vi "PPFS_TRAJECTORY_CMD_FIND_FOLLOW_SWERVE.vi"(6 "Pass_Through_Time":dbl=-1.0 format="%33.4f", 8 "Init":bool, 11 "Target Pose M":T1={"TRANSLATION"={"X"=0.0, "Y"=0.0}, "ROTATION"={"VALUE"=0.0, "COS"=1.0, "SIN"=0.0}} {"ROTATION"."SIN" format="%13.4f"; "ROTATION"."COS" format="%13.4f"; "ROTATION"."VALUE" format="%13.4f"; "TRANSLATION"."Y" format="%14.3f"; "TRANSLATION"."X" format="%14.3f"}) -> (0 "AtReference":bool, 1 "Complete":bool, 3 "Chassis Velocity Target SI":T4 {"vOmega" format="%10.3f"; "vY" format="%10.3f"; "vX" format="%10.3f"})   [LabVIEW 2019]
uses:
  <vilib>/Rock Robotics/WPI/ThirdParty/JAS_Junk/TrajLib/Trajectory_Library.lvlib
  PPFS_TRAJECTORY_GLOBALS.vi
  <vilib>/Rock Robotics/WPI/ThirdParty/MJansen/PathPlanner/PathPlanner24.lvlib
  <vilib>/Rock Robotics/WPI/ThirdParty/JAS_Junk/TrajLib/TypeDef/CHASSIS_SPEEDS.ctl
  <vilib>/Rock Robotics/WPI/ThirdParty/JAS_Junk/TrajLib/TypeDef/TRANSLATION2D.ctl
  <vilib>/Rock Robotics/WPI/ThirdParty/JAS_Junk/TrajLib/TypeDef/ROTATION2D.ctl
  <vilib>/Rock Robotics/WPI/ThirdParty/JAS_Junk/TrajLib/TypeDef/POSE2D.ctl
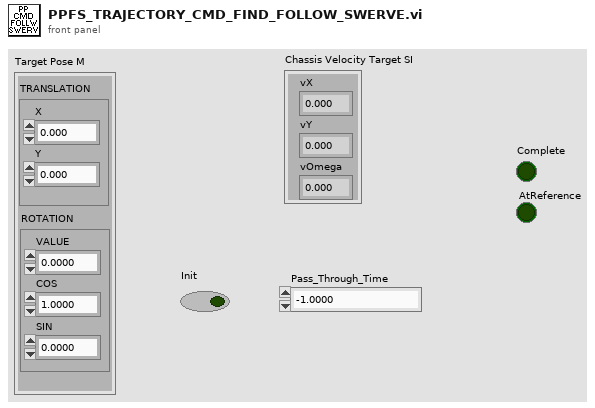
[diagram p1: front panel]
types:
  T1 = typedef "Trajectory_Library.lvlib/POSE2D.ctl" = cluster{"TRANSLATION":T2, "ROTATION":T3}
  T2 = typedef "Trajectory_Library.lvlib/TRANSLATION2D.ctl" = cluster{"X":dbl, "Y":dbl}
  T3 = typedef "Trajectory_Library.lvlib/ROTATION2D.ctl" = cluster{"VALUE":dbl, "COS":dbl, "SIN":dbl}
  T4 = typedef "Trajectory_Library.lvlib/CHASSIS_SPEEDS.ctl" = cluster{"vX":dbl, "vY":dbl, "vOmega":dbl}
  T5 = typedef "PathPlanner24.lvlib/PathPlannerPathConstraints.ctl" = cluster{"MaxVelocityMps;":dbl, "MaxAccelerationMpsSq;":dbl, "MaxAngularVelRadPsEc;":dbl, "MaxAngularAccRadPSecSq":dbl, "Exists":bool}
  T6 = typedef "Trajectory_Library.lvlib/PID_TUNING.ctl" = cluster{"Kp":dbl, "Ki":dbl, "Kd":dbl, "MaximumIntegral":dbl, "MinimumIntegral":dbl}
  T7 = typedef "Trajectory_Library.lvlib/PROFILED_PID_CONTROLLER.ctl" = cluster{"Controller":T8, "Goal":T9, "Setpoint":T9, "Constraint":T10}
  T8 = typedef "Trajectory_Library.lvlib/PID_CONTROLLER.ctl" = cluster{"Kp":dbl, "Ki":dbl, "Kd":dbl, "Period":dbl, "Max_Integral":dbl, "Min_Integral":dbl, "Max_Input":dbl, "Min_Input":dbl, "Continuous":bool, "PositionError":dbl, "VelocityError":dbl, "PrevError":dbl, "TotalError":dbl, "PositionTolerance":dbl, "VelocityTolerance":dbl, "SetPoint":dbl, "Kf":dbl, "Prev_Deriv":dbl, "Prev_Deriv 2":dbl, "DerivativeFilter":bool, "Min_Output":dbl, "Max_Output":dbl, "Prev_F_P":dbl, "Prev_F_P_2":dbl, "AntiWindupActive":bool, "Measurement":dbl}
  T9 = typedef "Trajectory_Library.lvlib/TRAPEZOID_PROFILE_STATE.ctl" = cluster{"Position":dbl, "Velocity":dbl}
  T10 = typedef "Trajectory_Library.lvlib/TRAPEZOID_PROFILE_CONSTRAINT.ctl" = cluster{"MaxVelocity":dbl, "MaxAcceleration":dbl}
  T11 = typedef "PathPlanner24.lvlib/PathPlannerReplanningConfig.ctl" = cluster{"enableInitialReplanning":bool, "enableDynamicReplanning":bool, "dynamicReplanningTotalErrorThreshold":dbl, "dynamicReplanningErrorSpikeThreshold":dbl}
  T12 = typedef "Trajectory_Library.lvlib/HOLONOMIC_PACK_TUNING.ctl" = cluster{"X PID Tuning":T6, "Y PID Tuning":T6, "thetaProfiledPID_CTRL":T7}
  T13 = typedef "PathPlanner24.lvlib/PathPlannerCmdFindConfig.ctl" = cluster{"Goal Position":T2, "GoalEndState":T14, "PathPlannerPathConstraints":T5, "Rotation Delay Distance M":dbl}
  T14 = typedef "PathPlanner24.lvlib/PathPlannerGoalEndState.ctl" = cluster{"Velocity":dbl, "Rotation":T3}
  T15 = typedef "PathPlanner24.lvlib/PathPlannerCmdFollowHolConfig.ctl" = cluster{"HOLONOMIC_CTRL_PACK_TUNING":T12, "Max Wheel Speed M/S":dbl, "Tolerance SI":T1, "Drive Base Radius M":dbl, "ControlPastEnd_Sec":dbl, "ReplanningConfig":T11, "Period_Sec":dbl, "Trigger Events":bool}
  T16 = typedef "Trajectory_Library.lvlib/HOLONOMIC_DRV_CTRL.ctl" = cluster{"poseTolerance":T1, "poseError":T1, "Enabled":bool, "PID_xCtrl":T8, "PID_yCtrl":T8, "PROF_PID_thetaCtrl":T7, "RotationError":T3, "FirstRun":bool}
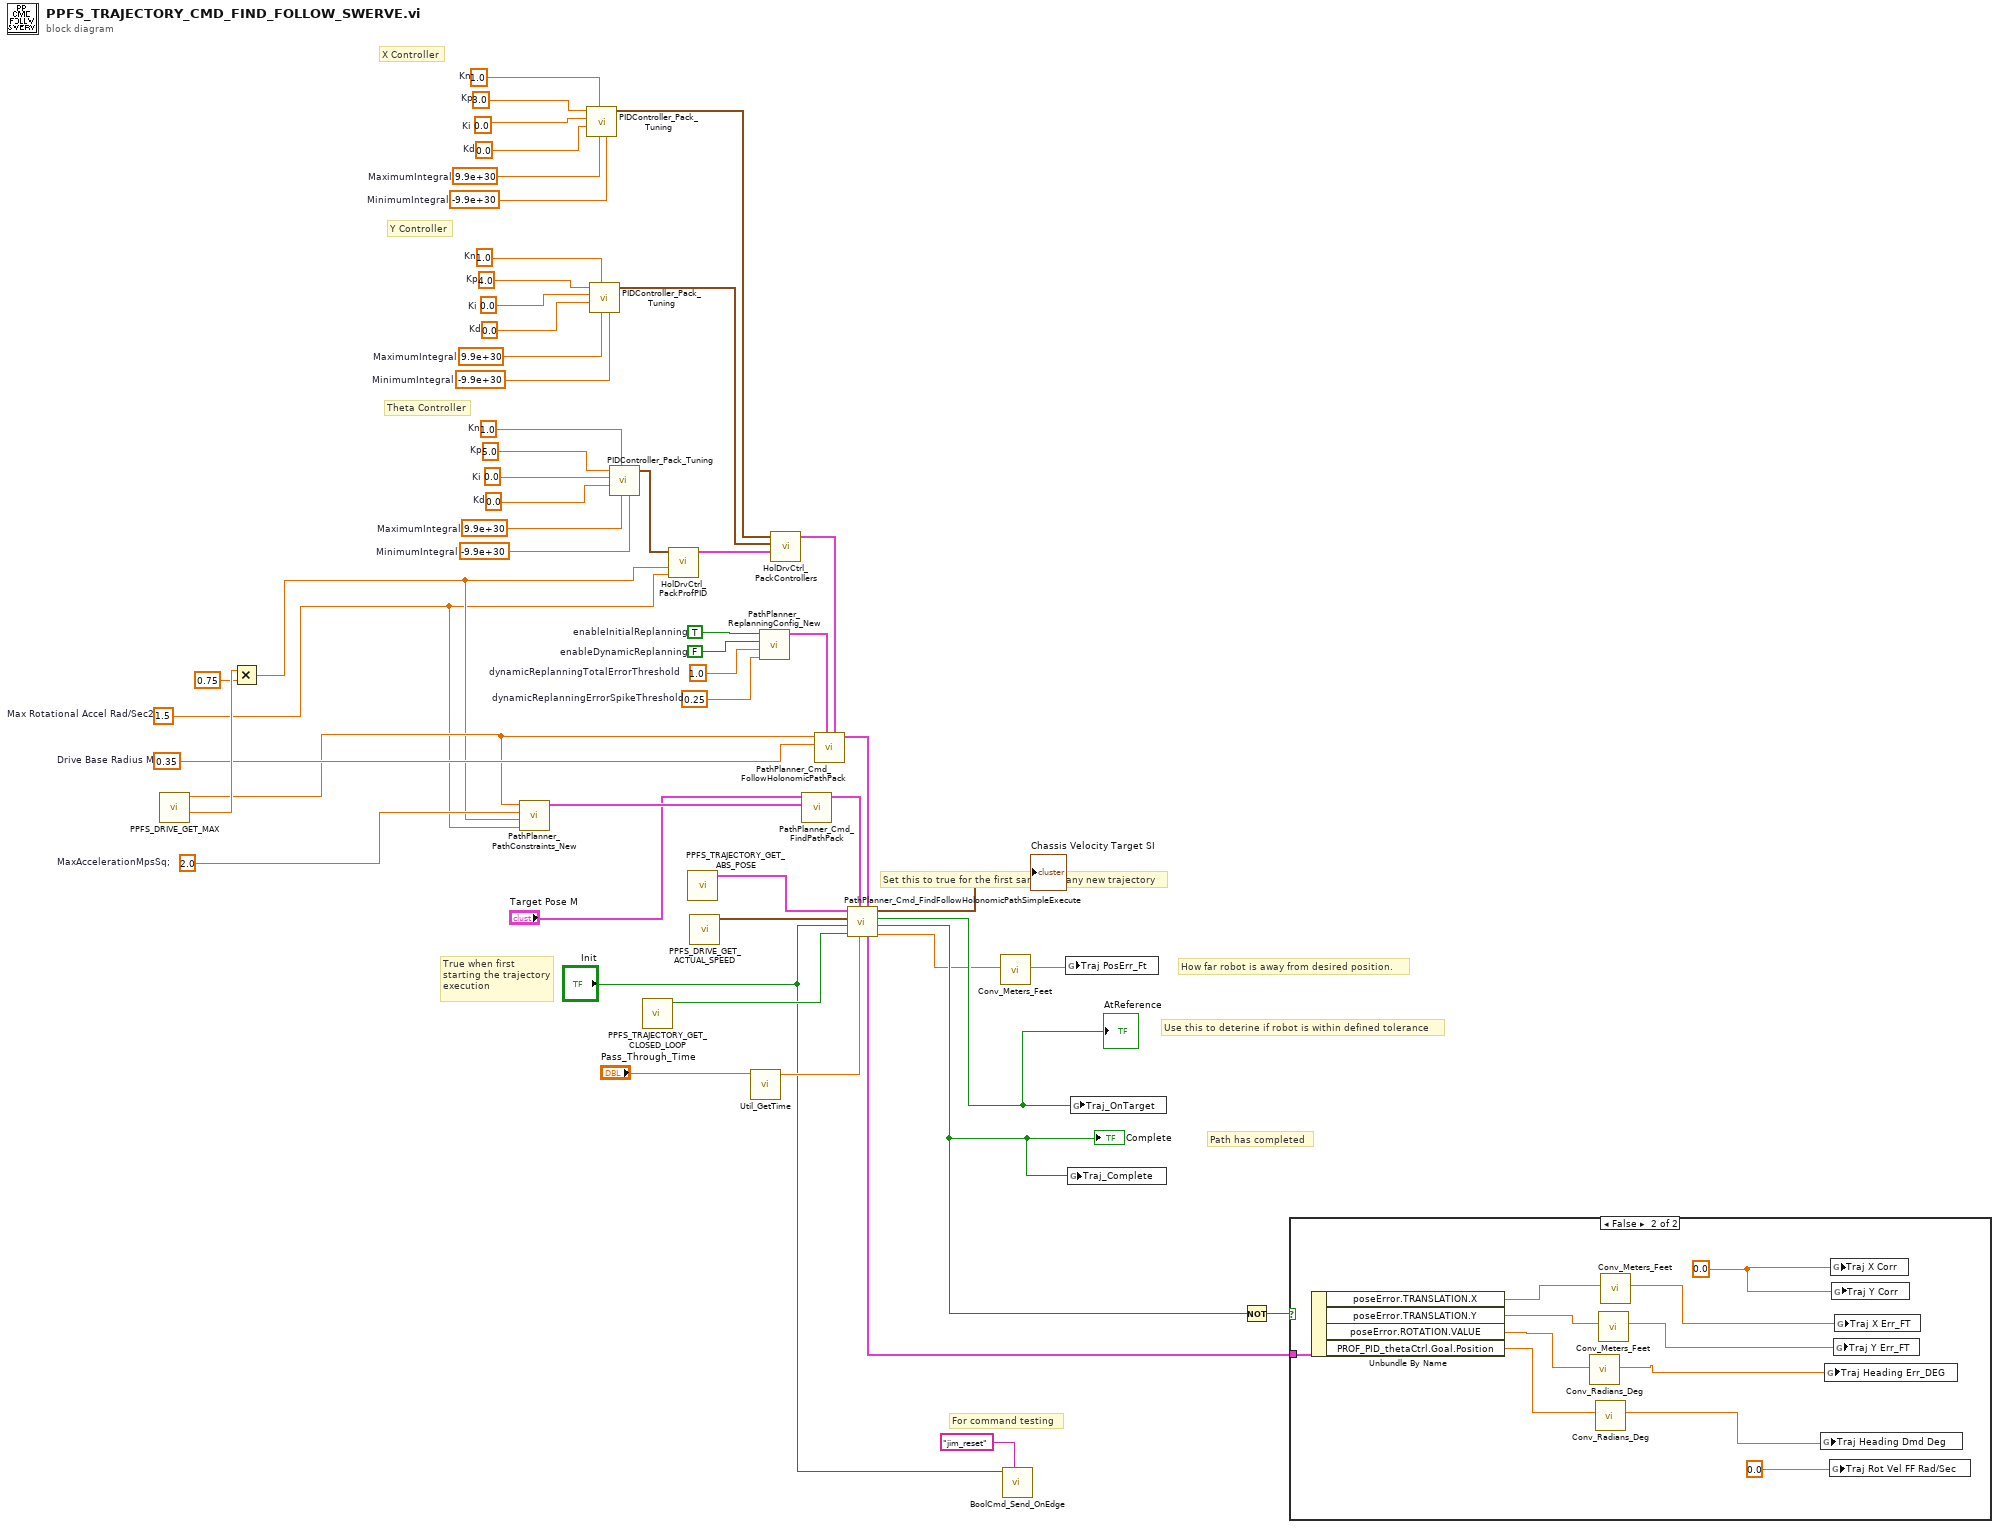
[diagram p0: block diagram]
diagram:
  w6 = 2.0  # MaxAccelerationMpsSq;
  w51 = TRUE  # enableInitialReplanning
  w50 = FALSE  # enableDynamicReplanning
  w49 = 1.0  # dynamicReplanningTotalErrorThreshold
  w48 = 0.25  # dynamicReplanningErrorSpikeThreshold
  w38 = 1.0  # Kn
  w35 = 5.0  # Kp
  w26 = 0.0  # Ki
  w25 = 0.0  # Kd
  w24 = 9.9e+30  # MaximumIntegral
  w23 = -9.9e+30  # MinimumIntegral
  w40 = 1.0  # Kn
  w37 = 3.0  # Kp
  w34 = 0.0  # Ki
  w33 = 0.0  # Kd
  w32 = 9.9e+30  # MaximumIntegral
  w31 = -9.9e+30  # MinimumIntegral
  w39 = 1.0  # Kn
  w36 = 4.0  # Kp
  w30 = 0.0  # Ki
  w29 = 0.0  # Kd
  w28 = 9.9e+30  # MaximumIntegral
  w27 = -9.9e+30  # MinimumIntegral
  w22 = 0.35  # Drive Base Radius M
  w1 = 1.5  # Max Rotational Accel Rad/Sec2
  # "Set this to true for the first sample of any new trajectory"
  # "For command testing"
  # "Path has completed"
  # "How far robot is away from desired position."
  # "Use this to deterine if robot is within defined tolerance"
  # "Theta Controller"
  # "Y Controller"
  # "X Controller"
  # "True when first\nstarting the trajectory\nexecution"
  n1 = call "PPFS_DRIVE_GET_MAX.vi"() -> ("Max Rotational Vel (Rad/Sec)"=w53:dbl, "Max Wheel Vel (Meter/Sec)"=w3:dbl)  [unwired: 10 in]
  n2 = Multiply(x=w53, y=0.75) -> (x*y=w2:dbl)
  n3 = call <vilib>:"PathPlanner_PathConstraints_New.vi"("MaxAngularAccRadPSecSq"=w1, "MaxAngularVelRadPsEc;"=w2, "MaxAccelerationMpsSq;"=w6, "MaxVelocityMps;"=w3) -> ("PathPlannerConstraints"=w7:T5)  [unwired: 7 in]
  n4 = call <vilib>:"PIDController_Pack_Tuning.vi"("MinimumIntegral"=w31, "MaximumIntegral"=w32, "Kn"=w40, "Kd"=w33, "Ki"=w34, "Kp"=w37) -> ("PID Tuning"=w44:T6)  [unwired: 5 in]
  n5 = call <vilib>:"PIDController_Pack_Tuning.vi"("MinimumIntegral"=w27, "MaximumIntegral"=w28, "Kn"=w39, "Kd"=w29, "Ki"=w30, "Kp"=w36) -> ("PID Tuning"=w45:T6)  [unwired: 5 in]
  n6 = call <vilib>:"PIDController_Pack_Tuning.vi"("MinimumIntegral"=w23, "MaximumIntegral"=w24, "Kn"=w38, "Kd"=w25, "Ki"=w26, "Kp"=w35) -> ("PID Tuning"=w41:T6)  [unwired: 5 in]
  n7 = call "PPFS_TRAJECTORY_GET_CLOSED_LOOP.vi"() -> ("AUTO_CLOSED_LOOP"=w19:bool)  [unwired: 11 in]
  n8 = call <vilib>:"HolDrvCtrl_PackProfPID.vi"("Max Accel"=w1, "Max Speed"=w2, "Theta PID Tuning"=w41) -> ("Theta PID CONTROLLER"=w46:T7)  [unwired: 8 in]
  n9 = call "PPFS_TRAJECTORY_GET_ABS_POSE.vi"() -> ("Absolute Odometry Pose"=w21:T1)  [unwired: 11 in]
  n10 = call "PPFS_DRIVE_GET_ACTUAL_SPEED.vi"() -> ("Drv Chassis Actual Velocity"=w20:T4)  [unwired: 11 in]
  n11 = call <vilib>:"Util_GetTime.vi"("Pass_Through_Time"="Pass_Through_Time") -> ("FPGA_Time_Seconds"=w17:dbl)  [unwired: 8 in, 2 out]
  n12 = call <vilib>:"PathPlanner_ReplanningConfig_New.vi"("dynamicReplanningErrorSpikeThreshold"=w48, "dynamicReplanningTotalErrorThreshold"=w49, "enableDynamicReplanning"=w50, "enableInitialReplanning"=w51) -> ("ReplanningConfig"=w47:T11)  [unwired: 7 in]
  n13 = call <vilib>:"HolDrvCtrl_PackControllers.vi"("thetaProfiledPID_CTRL"=w46, "Y PID Tuning"=w45, "X PID Tuning"=w44) -> ("HOLONOMIC_CTRL_PACK_TUNING"=w43:T12)  [unwired: 8 in]
  n14 = call <vilib>:"PathPlanner_Cmd_FindPathPack.vi"("PathPlannerPathConstraints"=w7, "Target Pose M"="Target Pose M") -> ("PathPlanner_Cmd_FindConfig"=w4:T13)  [unwired: 9 in]
  n15 = call <vilib>:"PathPlanner_Cmd_FollowHolonomicPathPack.vi"("HOLONOMIC_CTRL_PACK_TUNING"=w43, "ReplanningConfig"=w47, "Drive Base Radius M"=w22, "Max Wheel Speed M/S"=w3) -> ("PathPlanner_Ctrl_HolDrvConfig"=w42:T15)  [unwired: 7 in]
  n16 = call <vilib>:"PathPlanner_Cmd_FindFollowHolonomicPathSimpleExecute.vi"("PathPlanner_Cmd_FollowHolConfig"=w42, "PassthroughTime_SEC"=w17, "PathPlanner_Cmd_FindConfig"=w4, "Enabled"=w19, "Reset"="Init", "CurrentChassisSpeeds"=w20, "Current Pose SI"=w21) -> ("Position Error M"=w10:dbl, "Complete"=w12:bool, "At Reference"=w14:bool, "calcChassisSpeed"=→"Chassis Velocity Target SI":T4, "outHOLONOMIC_DRV_CTRL"=w15:T16)
  "AtReference" <- w14
  "Complete" <- w12
  n17 = call <vilib>:"Conv_Meters_Feet.vi"("Meters"=w10) -> ("Feet"=w11:dbl)  [unwired: 10 in]
  n18 = call <vilib>:"BoolCmd_Send_OnEdge.vi"("Command Name"="jim_reset", "Value"="Init") -> ()  [unwired: 9 in, 1 out]
  n19 = global write "PPFS_TRAJECTORY_GLOBALS.vi" "Traj PosErr_Ft"(w11) -> ()
  n20 = global write "PPFS_TRAJECTORY_GLOBALS.vi" "Traj_Complete"(w12) -> ()
  n21 = global write "PPFS_TRAJECTORY_GLOBALS.vi" "Traj_OnTarget"(w14) -> ()
  n22 = Not(x=w12) -> (.not. x?=w13:bool)
  n23 = case shown="False" w13 {
    tunnel: w15 -> [_ w60]
    frame True {
    }
    frame False {
      w64 = 0.0 ("Y Corr")
      n24 = Unbundle By Name(w60) -> ("poseError.TRANSLATION.X"=w59:dbl, "poseError.TRANSLATION.Y"=w58:dbl, "poseError.ROTATION.VALUE"=w57:dbl, "PROF_PID_thetaCtrl.Goal.Position"=w55:dbl)
      n25 = call <vilib>:"Conv_Radians_Deg.vi"("Radians"=w57) -> ("Degrees"=w56:dbl)  [unwired: 10 in]
      n26 = call <vilib>:"Conv_Radians_Deg.vi"("Radians"=w55) -> ("Degrees"=w54:dbl)  [unwired: 10 in]
      n27 = call <vilib>:"Conv_Meters_Feet.vi"("Meters"=w58) -> ("Feet"=w63:dbl)  [unwired: 10 in]
      n28 = call <vilib>:"Conv_Meters_Feet.vi"("Meters"=w59) -> ("Feet"=w62:dbl)  [unwired: 10 in]
      n29 = global write "PPFS_TRAJECTORY_GLOBALS.vi" "Traj Heading Dmd Deg"(w54) -> ()
      n30 = global write "PPFS_TRAJECTORY_GLOBALS.vi" "Traj Heading Err_DEG"(w56) -> ()
      n31 = global write "PPFS_TRAJECTORY_GLOBALS.vi" "Traj Rot Vel FF Rad/Sec"(0.0 ("Traj Heading Dmd Deg")) -> ()
      n32 = global write "PPFS_TRAJECTORY_GLOBALS.vi" "Traj X Corr"(w64) -> ()
      n33 = global write "PPFS_TRAJECTORY_GLOBALS.vi" "Traj Y Corr"(w64) -> ()
      n34 = global write "PPFS_TRAJECTORY_GLOBALS.vi" "Traj Y Err_FT"(w63) -> ()
      n35 = global write "PPFS_TRAJECTORY_GLOBALS.vi" "Traj X Err_FT"(w62) -> ()
    }
  }
